vi "solar_misc Get Bytes.vi"(8 "Old ByteOffset (0)":i32, 9 "Dimensions (0)":i32, 10 "ByteSize (0:STR,-1:PATH)":i32, 11 "ByteArray":u8[](array[numeric]) format="%.0x") -> (0 "New ByteOffset":i32, 2 "Value ByteSize":i32, 3 "Value ByteOffset":i32)   [LabVIEW 2018]
doc: "This returns the size of a string or path flattened data.\nStrings: <I32_size_prefix><data...>\nPaths: 'PTH0<I32_size_prefix><data...>"
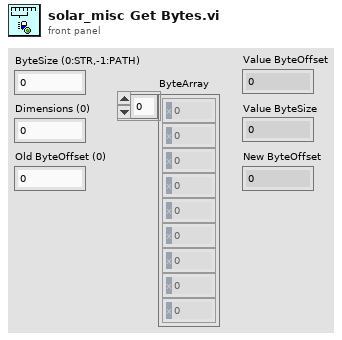
[diagram p1: front panel]
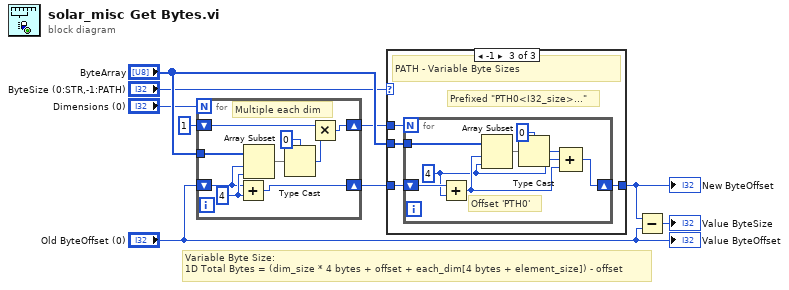
[diagram p0: block diagram]
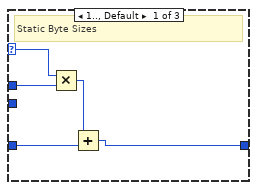
[diagram p2: hidden frame]
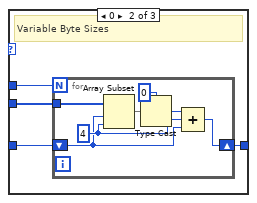
[diagram p3: hidden frame]
diagram:
  # "Variable Byte Size:\n1D Total Bytes = (dim_size * 4 bytes + offset + each_dim[4 bytes + element_size]) - offset"
  n1 = for {
    N: "Dimensions (0)" -> [_]
    tunnel: "ByteArray" -> [w18]
    shift-right: [w13] -> w3
    shift-left: "Old ByteOffset (0)" -> [w14]
    shift-right: [w11] -> w2
    shift-left: 1 -> [w10]
    w15 = 4 ("length")
    # "Multiple each dim"
    n2 = Add(x=w14, y=w15) -> (x+y=w13:i32)
    n3 = Array Subset(array=w18, index=w14, length=w15) -> (w17:u8[])
    n4 = Type Cast(type=0, x=w17) -> (*(type *) &x=w12:i32)
    n5 = Multiply(x=w10, y=w12) -> (x*y=w11:i32)
  }
  n6 = case shown="-1" "ByteSize (0:STR,-1:PATH)" {
    selector: "ByteSize (0:STR,-1:PATH)" -> [w22 _ _]
    tunnel: [w19 w27 w38] -> w8
    tunnel: w3 -> [w21 w26 w37]
    tunnel: w2 -> [w23 w25 w36]
    tunnel: "ByteArray" -> [_ w24 w35]
    frame 1.., Default {
      # "Static Byte Sizes"
      n7 = Multiply(x=w22, y=w23) -> (x*y=w20:i32)
      n8 = Add(x=w20, y=w21) -> (x+y=w19:i32)
    }
    frame 0 {
      # "Variable Byte Sizes"
      n9 = for {
        N: w25 -> [_]
        tunnel: w24 -> [w32]
        shift-right: [w28] -> w27
        shift-left: w26 -> [w29]
        w30 = 4 ("length")
        # "Add byte size of each element"
        n10 = Array Subset(array=w32, index=w29, length=w30) -> (w34:u8[])
        n11 = Type Cast(type=0 ("I32"), x=w34) -> (*(type *) &x=w31:i32)
        n12 = Compound Arithmetic op=ADD(w31, w30, w29) -> (w28:i32)
      }
    }
    frame -1 {
      # "Prefixed \"PTH0<I32_size>...\""
      # "PATH - Variable Byte Sizes"
      n13 = for {
        N: w36 -> [_]
        tunnel: w35 -> [w44]
        shift-right: [w42] -> w38
        shift-left: w37 -> [w41]
        w39 = 4 ("length")
        # "Offset 'PTH0'"
        # "Add byte size of each element"
        n14 = Add(x=w41, y=w39) -> (x+y=w40:i32)
        n15 = Array Subset(array=w44, index=w40, length=w39) -> (w46:u8[])
        n16 = Type Cast(type=0 ("I32"), x=w46) -> (*(type *) &x=w43:i32)
        n17 = Compound Arithmetic op=ADD(w43, w39, w40) -> (w42:i32)
      }
    }
  }
  "New ByteOffset" <- w8
  n18 = Subtract(x=w8, y="Old ByteOffset (0)") -> (x-y=→"Value ByteSize":i32)
  "Value ByteOffset" <- "Old ByteOffset (0)"
